vi "Close Stream.vi"(8 "error in (no error)":errorcluster, 11 "Channel GEI in":refnum<class "Channel.lvclass">) -> (0 "error out":errorcluster, 3 "Channel GEI out":refnum<class "Channel.lvclass">)   [LabVIEW 2018, in "Channel.lvclass"]
uses:
  Channel.lvclass
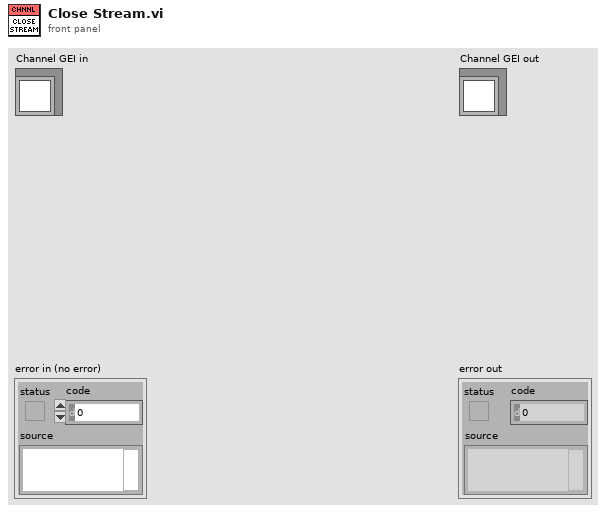
[diagram p1: front panel]
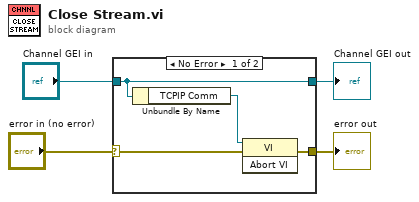
[diagram p0: block diagram]
diagram:
  n1 = case shown="No Error" "error in (no error)" {
    selector: "error in (no error)" -> [w6 w10]
    tunnel: [w5 w10] -> w3
    tunnel: [w8 w9] -> w1
    tunnel: "Channel GEI in" -> [w8 w9]
    frame No Error {
      n2 = Unbundle By Name(w8) -> ("TCPIP Comm"=w7:refnum<vi>)
      n3 = invoke class="VI" method="Abort VI"(reference=w7, error in=w6) -> (error out=w5:errorcluster)  [unwired: 1 in, 2 out]
    }
    frame Error {
    }
  }
  "error out" <- w3
  "Channel GEI out" <- w1
